vi "TeslaVelox_GlobalConfig.vi"() -> ()   [LabVIEW 2018, in "TeslaVeloxProbeStation.lvclass"]
uses:
  TeslaVeloxProbeStation.lvclass
panel:
  in  "Tesla Probestation configuration":T1={"IP address"="192.168.1.10", "Separation gap[um]"=500.0, "Port Number"=1412, "Use Overdrive?"=FALSE, "Touchdown method"=enum."no feedback", "Coordinate system"=enum."X as index"}
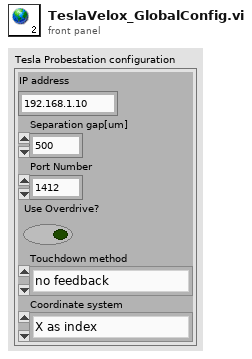
[diagram p1: front panel]
types:
  T1 = cluster{"IP address":string, "Separation gap[um]":dbl, "Port Number":i32, "Use Overdrive?":bool, "Touchdown method":enum16{"no feedback"}, "Coordinate system":enum16{"Cartesian", "X as index"}}
diagram:
